vi "freshHold.vi"() -> ()   [LabVIEW 2016]
panel:
  in  "fresh hold":dbl
  out "TRIGGERED":bool
  in  "Slide":dbl(slide) scale=0.0..10.0
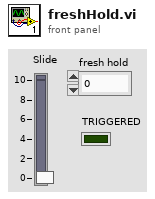
[diagram p1: front panel]
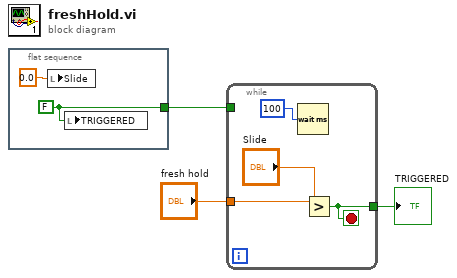
[diagram p0: block diagram]
diagram:
  n1 = flat-sequence {
    tunnel: [w4] -> w1
    frame #0 {
      w4 = FALSE
      n2 = local write "Slide"(0.0) -> ()
      n3 = local write "TRIGGERED"(w4) -> ()
    }
  }
  n4 = while {
    tunnel: "fresh hold" -> [w6]
    tunnel: [w9] -> w2
    tunnel: w1 -> [_]
    stop <- w9 stop-if-true
    n5 = Wait (ms)(milliseconds to wait=100) -> ()  [unwired: 1 out]
    n6 = Greater?(x="Slide", y=w6) -> (0:w9:bool)
  }
  "TRIGGERED" <- w2
